vi "Punkte_mit_linie_verbinden_tracking.vi"(6 "Color":u32, 8 "Boolean":bool, 9 "Array":dbl[][](array[numeric]), 10 "dimension size":i32, 11 "Refnum in":T1) -> (3 "Refnum out":T1)   [LabVIEW 2014]
uses:
  <vilib>/vision/Image Controls.llb/IMAQ Image.ctl
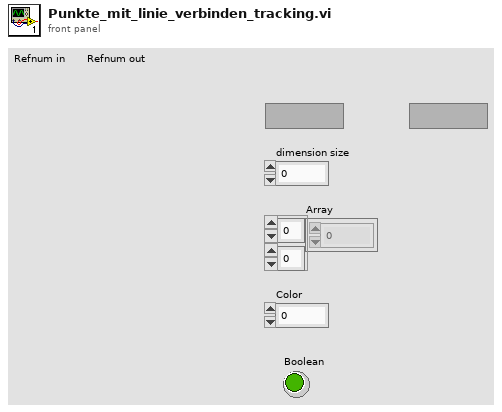
[diagram p1: front panel]
types:
  T1 = typedef "IMAQ Image.ctl" = refnum<image>
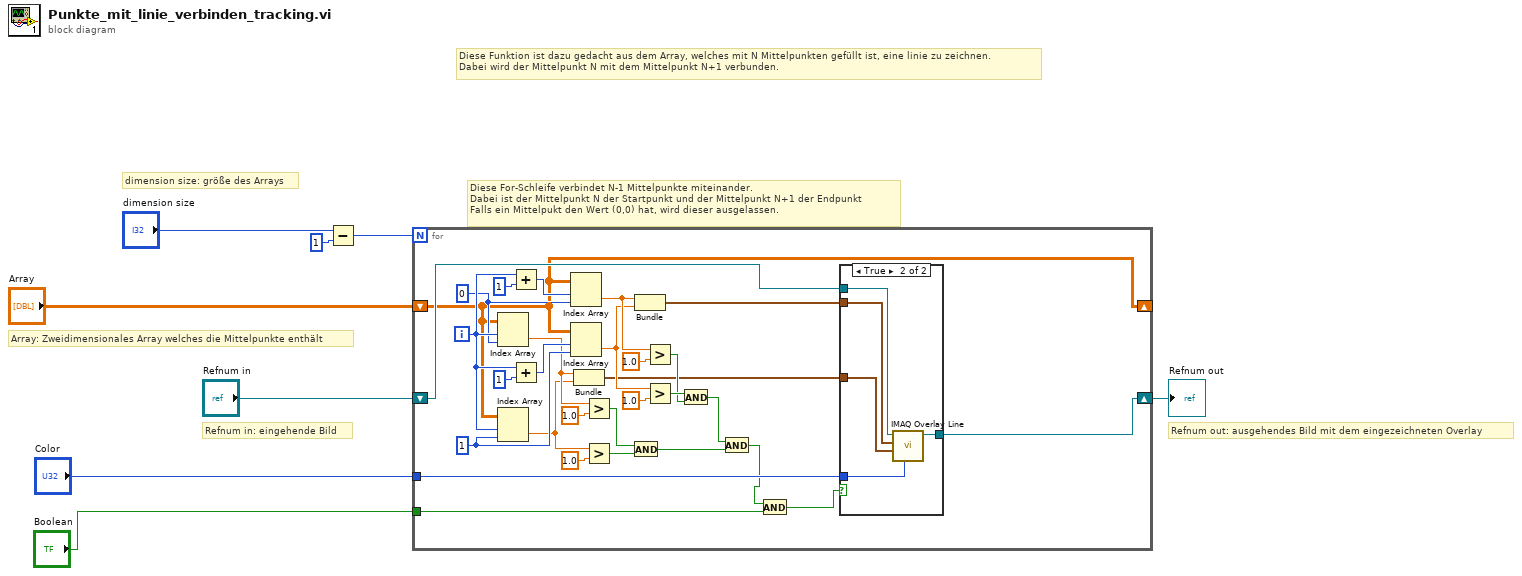
[diagram p0: block diagram]
diagram:
  # "Diese For-Schleife verbindet N-1 Mittelpunkte miteinander. \nDabei ist der Mittelpunkt N der Startpunkt und der Mittelpunkt N+1 der Endpunkt\nFalls ein Mittelpukt den Wert (0,0) hat, wird dieser ausgelassen."
  # "Refnum out: ausgehendes Bild mit dem eingezeichneten Overlay"
  # "Refnum in: eingehende Bild"
  # "Array: Zweidimensionales Array welches die Mittelpunkte enthält"
  # "dimension size: größe des Arrays"
  # "Diese Funktion ist dazu gedacht aus dem Array, welches mit N Mittelpunkten gefüllt ist, eine linie zu zeichnen. \nDabei wird der Mittelpunkt N mit dem Mittelpunkt N+1 verbunden."
  n1 = Subtract(x="dimension size", y=1) -> (x-y=w5:i32)
  n2 = for {
    N: w5 -> [_]
    shift-right: [w14] -> _
    shift-left: "Array" -> [w14]
    shift-right: [w38] -> w3
    shift-left: "Refnum in" -> [w37]
    tunnel: "Color" -> [w15]
    tunnel: "Boolean" -> [w10]
    i -> [w36]
    w32 = 0 ("index (col)")
    w33 = 1 ("disabled index (col)")
    n3 = Index Array(array=w14, index (row)=w36, index (col)=w32) -> (element=w19:dbl)
    n4 = Index Array(array=w14, index (row)=w36, index (col)=w33) -> (element=w18:dbl)
    n5 = Add(x=w36, y=1) -> (x+y=w35:i32)
    n6 = Add(x=w36, y=1) -> (x+y=w34:i32)
    n7 = Index Array(array=w14, index (row)=w35, index (col)=w32) -> (element=w25:dbl)
    n8 = Index Array(array=w14, index (row)=w34, index (col)=w33) -> (element=w24:dbl)
    n9 = Bundle("element"=w19, "element"=w18) -> (w12:cluster{"element":dbl, "element":dbl})  [unwired: 1 in]
    n10 = Greater?(x=w19, y=1.0) -> (0:w21:bool)
    n11 = Greater?(x=w18, y=1.0) -> (0:w20:bool)
    n12 = And(x=w21, y=w20) -> (x .and. y?=w16:bool)
    n13 = Bundle("element"=w25, "element"=w24) -> (w13:cluster{"element":dbl, "element":dbl})  [unwired: 1 in]
    n14 = Greater?(x=w25, y=1.0) -> (0:w26:bool)
    n15 = Greater?(x=w24, y=1.0) -> (0:w27:bool)
    n16 = And(x=w27, y=w26) -> (x .and. y?=w17:bool)
    n17 = And(x=w17, y=w16) -> (x .and. y?=w11:bool)
    n18 = And(x=w11, y=w10) -> (x .and. y?=w9:bool)
    n19 = case shown="True" w9 {
      tunnel: [w39 w44] -> w38
      tunnel: w37 -> [w39 w43]
      tunnel: w12 -> [_ w40]
      tunnel: w13 -> [_ w41]
      tunnel: w15 -> [_ w42]
      frame False {
      }
      frame True {
        n20 = call "IMAQ Overlay Line"("Color"=w42, "End Point"=w40, "Start Point"=w41, "Image"=w43) -> ("Image Out"=w44:T1)  [unwired: 6 in, 1 out]
      }
    }
  }
  "Refnum out" <- w3
